vi "Create Message.vi"(2 "cmd":T2, 3 "data":variant) -> (4 "msg":T1)   [LabVIEW 2021, in "Seq Edit Quick Drop.lvlib"]
uses:
  Seq Edit Quick Drop.lvlib
  Command.ctl
  Message.ctl
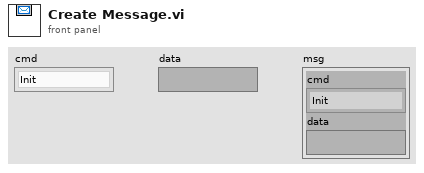
[diagram p1: front panel]
types:
  T1 = typedef "Seq Edit Quick Drop.lvlib/Message.ctl" = cluster{"cmd":T2, "data":variant}
  T2 = typedef "Seq Edit Quick Drop.lvlib/Command.ctl" = enum16{"Init", "Get Application Manager", "Shortcut Activated", "Display Tools", "Tool Selected", "Timeout", "Error", "Close"}
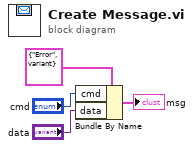
[diagram p0: block diagram]
diagram:
  n1 = Bundle By Name(cluster=T1 {"cmd"=enum."Error", "data"=variant} ("cmd"), "cmd"="cmd", "data"="data") -> (→"msg":T1)
